vi "SearchKey.vi"(5 "In":string, 12 "KEY1":string, 13 "KEY2":string) -> (6 "Data":string[](array[string]), 8 "String":string, 10 "Position":i32)   [LabVIEW 2017]
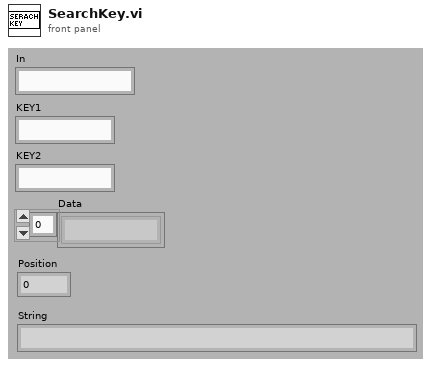
[diagram p1: front panel]
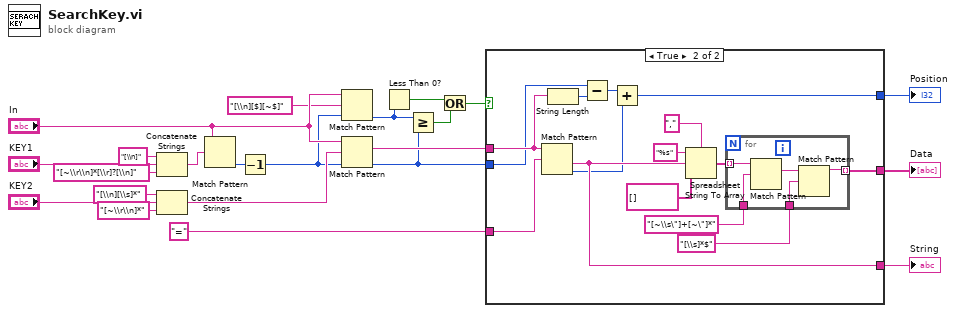
[diagram p0: block diagram]
diagram:
  n1 = Concatenate Strings("[\\n]" ("string"), "KEY1", "[~\\r\\n]*[\\r]?[\\n]" ("string")) -> (w21:string)
  n2 = Concatenate Strings("[\\n][\\s]*" ("string"), "KEY2", "[~\\r\\n]*" ("string")) -> (w13:string)
  n3 = Match Pattern(string="In", regular expression=w21) -> (offset past match=w12:i32)  [unwired: 4 out]
  n4 = Decrement(x=w12) -> (x-1=w6:i32)
  n5 = Match Pattern(string="In", regular expression="[\\n][$][~$]" ("string"), offset (0)=w6) -> (offset past match=w4:i32)  [unwired: 3 out]
  n6 = Match Pattern(string="In", regular expression=w13, offset (0)=w6) -> (match substring=w11:string, offset past match=w5:i32)  [unwired: 2 out]
  n7 = Less Than 0?(x=w4) -> (x < 0?=w3:bool)
  n8 = Greater Or Equal?(x=w4, y=w5) -> (x >= y?=w2:bool)
  n9 = Or(x=w3, y=w2) -> (x .or. y?=w1:bool)
  n10 = case shown="TRUE" w1 {
    tunnel: "=" ("regular expression") -> [_ w36]
    tunnel: [_ w35] -> w15
    tunnel: [_ w32] -> w14
    tunnel: w11 -> [_ w30]
    tunnel: [_ w26] -> w10
    tunnel: w5 -> [_ w23]
    frame False {
    }
    frame True {
      n11 = Match Pattern(string=w30, regular expression=w36) -> (after substring=w35:string, offset past match=w28:i32)  [unwired: 3 out]
      n12 = String Length(string=w30) -> (length=w29:i32)
      n13 = Subtract(x=w23, y=w29) -> (x-y=w27:i32)
      n14 = Add(x=w27, y=w28) -> (x+y=w26:i32)
      n15 = Spreadsheet String To Array(delimiter (Tab)=",", format string="%s", spreadsheet string=w35, array type (2D Dbl)=string[] []) -> (array=w31:string[])
      n16 = for {
        tunnel: w31 -> [w41] mode=indexing
        tunnel: [w38] -> w32 mode=indexing
        tunnel: "[~\\s\"]+[~\"]*" ("regular expression") -> [w40]
        tunnel: "[\\s]*$" ("regular expression") -> [w39]
        n17 = Match Pattern(string=w41, regular expression=w40) -> (match substring=w42:string)  [unwired: 4 out]
        n18 = Match Pattern(string=w42, regular expression=w39) -> (before substring=w38:string)  [unwired: 4 out]
      }
    }
  }
  "Data" <- w14
  "Position" <- w10
  "String" <- w15
